vi "IHM_CloseLauncher.vi"(8 "error in (no error)":errorcluster, 11 "VI reference":refnum<vi>) -> (0 "error out":errorcluster)   [LabVIEW 2013]
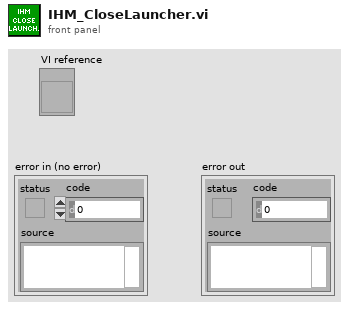
[diagram p1: front panel]
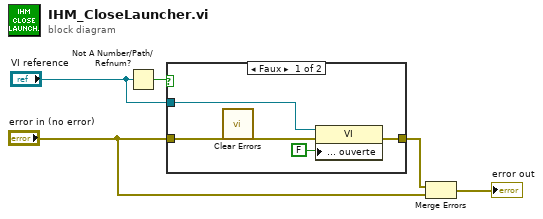
[diagram p0: block diagram]
diagram:
  n1 = Not A Number/Path/Refnum?(number/path/refnum="VI reference") -> (NaN/Path/Refnum?=w5:bool)
  n2 = case shown="Faux" w5 {
    tunnel: "error in (no error)" -> [w7 w11]
    tunnel: [w10 w11] -> w4
    tunnel: "VI reference" -> [w8 _]
    frame False {
      n3 = call <vilib>:"Clear Errors.vi"("error in (no error)"=w7) -> ("error out"=w6:errorcluster)  [unwired: 6 out]
      n4 = property class="VI"(reference=w8, error in=w6, "Fenêtre face-avant : ouverte"=FALSE ("Front Panel Window:Open")) -> (error out=w10:errorcluster)  [unwired: 1 out]
    }
    frame True {
    }
  }
  n5 = Merge Errors(w4, "error in (no error)") -> (→"error out":errorcluster)
